vi "Do.vi"(8 "error in (no error)":errorcluster, 10 "Actor in":refnum<class "Actor.lvclass">, 11 "Flush Sequncer Msg":refnum<class "Flush Sequncer Msg.lvclass">) -> (0 "error out":errorcluster, 2 "Actor out":refnum<class "Actor.lvclass">)   [LabVIEW 2020, in "Sequencer.lvlib" / "Flush Sequncer Msg.lvclass"]
doc: "Flush the Sequencer Core message queue and clear the Interrupt Notifier and then release the Status Notifier to signal that the Flush was completed."
uses:
  Flush Sequncer Msg.lvclass
  PPL/HDH.Actor Framework.Core.Actor.lvlibp/1abvi3w/vi.lib/ActorFramework/Actor/Actor.lvclass
  Sequencer/Sequencer.lvclass
  C:/Current projects/WS/PPL/HDH.Actor Framework.Core.Actor.lvlibp/1abvi3w/vi.lib/ActorFramework/Actor/Actor.lvclass
  Flush Sequncer Msg.lvclass/Flush Sequncer Msg.ctl
  Sequencer/Sequencer.lvclass/Sequencer.ctl
  Sequencer Core/Sequencer Core.lvclass/Sequencer Core.ctl
  PPL/HDH.Data.Generic.lvlibp/Synchronization/Notifier/Cancel.vi
  Message Priority Queue/Flush.vi
  PPL/HDH.Data.Generic.lvlibp/Synchronization/Notifier/Notifier.lvclass
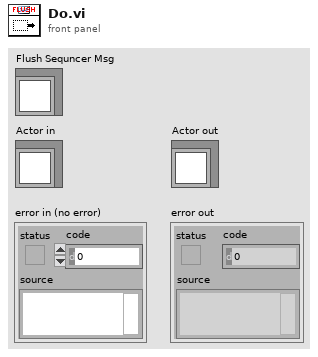
[diagram p1: front panel]
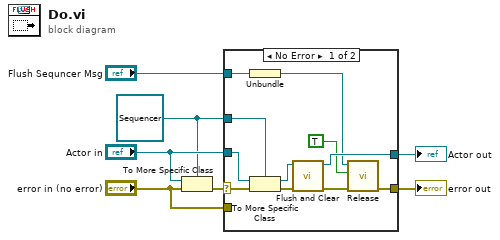
[diagram p0: block diagram]
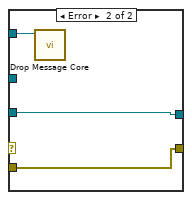
[diagram p2: hidden frame]
diagram:
  w1 = refnum<class "Sequencer.lvclass"> refnum ("Sequencer.lvlib:Sequencer.lvclass")
  n1 = To More Specific Class(target class=w1, reference="Actor in", error in="error in (no error)") -> (error out=w7:errorcluster)  [unwired: 1 out]
  n2 = case shown="No Error" w7 {
    selector: w7 -> [w18 _]
    tunnel: "Flush Sequncer Msg" -> [w12 w21]
    tunnel: [w9 w20] -> w5
    tunnel: "error in (no error)" -> [_ w20]
    tunnel: [w13 w19] -> w3
    tunnel: "Actor in" -> [w17 w19]
    tunnel: w1 -> [w16 _]
    frame No Error {
      n3 = Unbundle(w12) -> (w11:refnum<class "Notifier.lvclass">)
      n4 = To More Specific Class(target class=w16, reference=w17, error in=w18) -> (specific class reference=w15:refnum<class "Sequencer.lvclass">, error out=w14:errorcluster)
      n5 = call "Flush and Clear.vi"("error in (no error)"=w14, "Sequencer in"=w15) -> ("error out"=w10:errorcluster, "Sequencer out"=w13:refnum<class "Sequencer.lvclass">)  [unwired: 8 in]
      n6 = call "Release.vi"("error in (no error)"=w10, "Force destroy? (F)"=TRUE, "Notifier in"=w11) -> ("error out"=w9:errorcluster)  [unwired: 6 in, 2 out]
    }
    frame Error {
      n7 = call-dynamic "Drop Message Core.vi"("Flush Sequncer Msg in"=w21) -> ()  [unwired: 11 in]
    }
  }
  "error out" <- w5
  "Actor out" <- w3
